vi "Read Single I16 Image and Metadata from file.vi"(7 "File":refnum<file>, 8 "error out":errorcluster, 9 "Tags":T2[](array[typedef]), 10 "Litt/BigEnd":bool, 11 "Image":T1) -> (0 "error out":errorcluster, 3 "Image (duplicate)":T1, 5 "File dup":refnum<file>)   [LabVIEW 2015, in "Tiff reader.lvlib"]
doc: "Read a single image and it's metadata from a file ref."
uses:
  Tiff reader.lvlib
  FieldTypes.ctl
  IFD Entry.ctl
  <vilib>/vision/Image Controls.llb/IMAQ Image.ctl
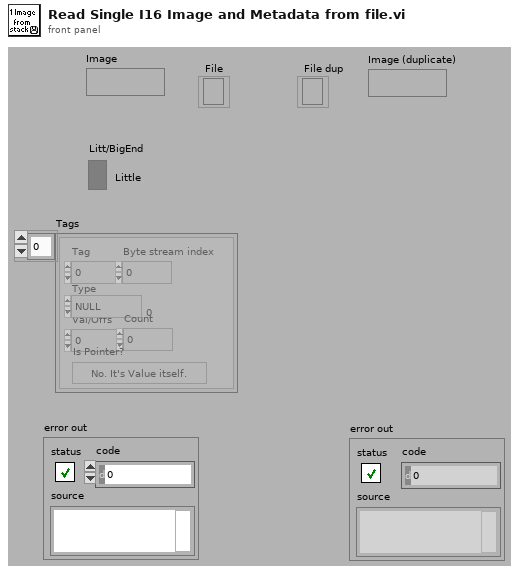
[diagram p1: front panel]
types:
  T1 = typedef "IMAQ Image.ctl" = refnum<image>
  T2 = typedef "Tiff reader.lvlib/IFD Entry.ctl" = cluster{"Tag":u16, "Type":T3, "Count":u32, "Val/Offs":u32, "Is Pointer?":bool, "Byte stream index":i32}
  T3 = typedef "Tiff reader.lvlib/FieldTypes.ctl" = enum16{"NULL", "U8", "ASCII7", "U16", "U32", "RATIONAL", "SByte(I8)", "Undef(8Bit)", "I16", "I32", "SRat(4B:4B)", "SGL(4Byte)", "DBL(8Byte)"}
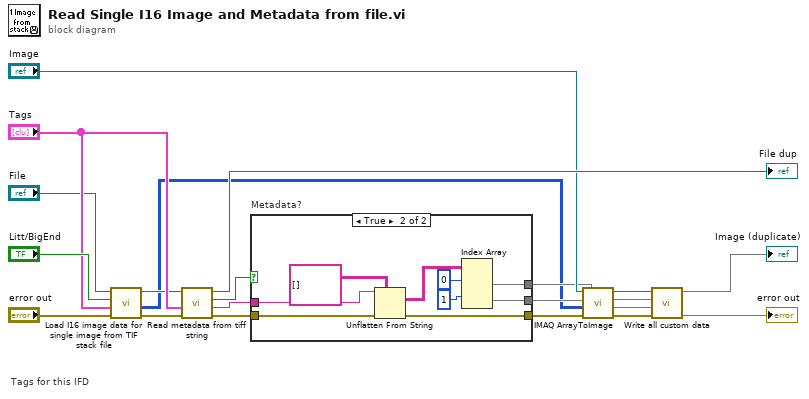
[diagram p0: block diagram]
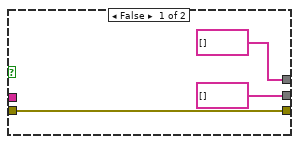
[diagram p2: hidden frame]
diagram:
  # "Tags for this IFD"
  n1 = call "Load I16 image data for single image from TIF stack file.vi"("error in"="error out", "DirEntries"="Tags", "Litt/BigEnd"="Litt/BigEnd", "File"="File") -> ("error out"=w10:errorcluster, "Gray16"=w1:i16[][], "File"=w9:refnum<file>)  [unwired: 5 out]
  n2 = call "Read metadata from tiff string.vi"("error in"=w10, "DirEntries"="Tags", "Tiff image stack"=w9) -> ("error out"=w12:errorcluster, "Metadata string"=w11:string, "Tag exists?"=w13:bool, "Tiff image stack dup"=→"File dup":refnum<file>)  [unwired: 1 in, 4 out]
  n3 = case "Metadata?" shown="True" w13 {
    tunnel: w11 -> [_ w31]
    tunnel: w12 -> [w22 w29]
    tunnel: [string[] [] w27] -> w6
    tunnel: [string[] [] w26] -> w8
    tunnel: [w22 w23] -> w17
    frame False {
    }
    frame True {
      n4 = Unflatten From String(type=string[][] [], binary string=w31, error in (no error)=w29) -> (value=w28:string[][], error out=w23:errorcluster)  [unwired: 3 out]
      n5 = Index Array(array=w28, index (row) #1=0 ("index (row)"), index (row) #2=1 ("index (row)")) -> (element #1=w27:string[], element #2=w26:string[])  [unwired: 2 in]
    }
  }
  n6 = call "IMAQ ArrayToImage"("error in (no error)"=w17, "Image Pixels (I16)"=w1, "Image"="Image") -> ("error out"=w5:errorcluster, "Image Out"=w2:T1)  [unwired: 3 in, 4 out]
  n7 = call "Write all custom data.vi"(8:w5, 9:w8, 10:w6, 11:w2) -> (0:→"error out", 3:→"Image (duplicate)")  [unwired: 6 out]
